vi "WriteToServo.vi"(9 "Position":u8, 10 "Servo":enum16{"Base", "Arm", "Wrist", "Grip"}(ring), 11 "VISA resource name":refnum<visa-resource-name>) -> (3 "VISA resource name out":refnum<visa-resource-name>)   [LabVIEW 2014]
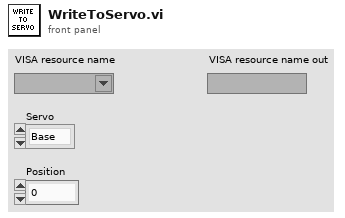
[diagram p1: front panel]
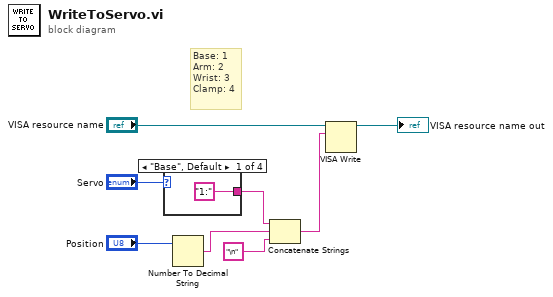
[diagram p0: block diagram]
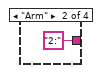
[diagram p2: hidden frame]
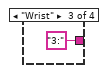
[diagram p3: hidden frame]
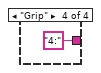
[diagram p4: hidden frame]
diagram:
  # "Base: 1\nArm: 2\nWrist: 3\nClamp: 4"
  n1 = case shown="\"Base\", Default" "Servo" {
    tunnel: ["1:" "2:" "3:" "4:"] -> w4
    frame "Base", Default {
    }
    frame "Arm" {
    }
    frame "Wrist" {
    }
    frame "Grip" {
    }
  }
  n2 = Number To Decimal String(number="Position") -> (decimal integer string=w8:string)  [unwired: 1 in]
  n3 = Concatenate Strings(w4, w8, "\n") -> (w1:string)
  n4 = VISA Write(VISA resource name="VISA resource name", write buffer=w1) -> (VISA resource name out=→"VISA resource name out":refnum<visa-resource-name>)  [unwired: 1 in, 2 out]
